vi "HFRR ADV v09.vi"() -> ()   [LabVIEW 2025] (continued)
                    n430 = local write "Main Dashboard Buttons"(T1."Home" ("Main Dashboard Buttons")) -> ()
                  }
                }
              }
              frame "Calibrate" {
              }
            }
          }
          frame #2 {
            n431 = Not(x=w709) -> (.not. x?=w708:bool)
            n432 = local write "Confirm Measrurement"(w708) -> ()
            n433 = local read "Calibration Tab"() -> (w707:enum32{"Measrument", "Calibrate"})
            n434 = case shown="\"Measrument\", Default" w707 {
              frame "Measrument", Default {
                n435 = local write "Main Tab"(T2."HOME" ("Main Tab")) -> ()
              }
              frame "Calibrate" {
              }
            }
          }
        }
      }
    }
    n436 = local read "Humidity"() -> (w462:bool)
    n437 = local read "Save Change"() -> (w467:bool)
    n438 = local read "Calibrate"() -> (w468:bool)
    n439 = local read "Auto Start Test"() -> (w463:bool)
    n440 = case shown="True" w468 {
      selector: w468 -> [_ w575]
      frame False {
      }
      frame True {
        n441 = Not(x=w575) -> (.not. x?=w574:bool)
        n442 = local write "Calibrate"(w574) -> ()
        n443 = local write "Calibration Tab"(enum32{"Measrument", "Calibrate"}."Calibrate" ("Calibration Tab")) -> ()
      }
    }
    n444 = case shown="True" w467 {
      selector: w467 -> [_ w519]
      frame False {
      }
      frame True {
        n445 = stacked-sequence {
          tunnel: w519 -> [_ _ _ _ w573]
          frame #0 {
            n446 = call "IMAGE ANALYSIS.vi"("Enum"=POST_ANALYSIS_ENUM."HIDE UI") -> ()  [unwired: 9 in, 2 out]
          }
          frame #1 {
            n447 = local read "100x gain"() -> (w521:dbl)
            n448 = local read "10x Gain"() -> (w522:dbl)
            n449 = local read "5x Gain"() -> (w523:dbl)
            n450 = Number To Fractional String(number=w522, width (-)=i16 4, precision (6)=i16 7) -> (F-format string=w544:string)  [unwired: 1 in]
            n451 = Number To Fractional String(number=0.0, width (-)=i16 4, precision (6)=i16 7) -> (F-format string=w539:string)  [unwired: 1 in]
            n452 = Number To Fractional String(number=w521, width (-)=i16 4, precision (6)=i16 7) -> (F-format string=w527:string)  [unwired: 1 in]
            n453 = Number To Fractional String(number=w523, width (-)=i16 10 ("precision (6)"), precision (6)=i16 7) -> (F-format string=w553:string)  [unwired: 1 in]
            n454 = Concatenate Strings("[CH1]" ("string"), w553, " - 5x Gain" ("string"), "\r") -> (w543:string)
            n455 = Concatenate Strings("[CH2]" ("string"), w544, " - 10x Gain" ("string"), "\r") -> (w542:string)
            n456 = Concatenate Strings("[CH3]" ("string"), w539, " - 20x Gain" ("string"), "\r") -> (w533:string)
            n457 = Concatenate Strings("[CH4]" ("string"), w527, " - 100x Gain" ("string"), "\r") -> (w526:string)
            n458 = String To Path(string="C:\\LAB-IQ\\Image Calibrate v01.dcf") -> (path=w556:path)
            n459 = Concatenate Strings(w543, w542, w533, w526) -> (w541:string)
            n460 = call <vilib>:"Write Characters To File.vi"("append to file? (new file:F)"=FALSE, "character string"=w541, "file path (dialog if empty)"=w556) -> ()  [unwired: 2 in, 1 out]
          }
          frame #2 {
            n461 = String To Path(string="C:\\LAB-IQ\\Image Calibrate v01.dcf") -> (path=w559:path)
            n462 = Open/Create/Replace File ("Open File")(file path (use dialog)=w559) -> (refnum out=w560:refnum<file>)  [unwired: 5 in, 2 out]
            n463 = for {
              N: 4 -> [_]
              tunnel: w560 -> [w566]
              i -> [w562]
              n464 = Read from Text File ("Read File")(file (use dialog)=w566) -> (text=w567:string)  [unwired: 3 in, 3 out]
              n465 = String Subset(string=w567, offset (0)=6, length (rest)=10 ("length (rest)")) -> (substring=w563:string)
              n466 = Fract/Exp String To Number(string=w563) -> (number=w561:dbl)  [unwired: 3 in, 1 out]
              n467 = case shown="3" w562 {
                tunnel: w561 -> [w568 w569 _ w570 _]
                frame 0 {
                  n468 = local write "5x Gain"(w568) -> ()
                }
                frame 1 {
                  n469 = local write "10x Gain"(w569) -> ()
                }
                frame 2 {
                }
                frame 3 {
                  n470 = local write "100x gain"(w570) -> ()
                }
                frame 4, Default {
                }
              }
            }
          }
          frame #3 {
            n471 = call "IMAGE ANALYSIS.vi"("Enum"=POST_ANALYSIS_ENUM."SHOW UI") -> ()  [unwired: 9 in, 2 out]
          }
          frame #4 {
            n472 = Not(x=w573) -> (.not. x?=w572:bool)
            n473 = local write "Save Change"(w572) -> ()
          }
        }
      }
    }
    n474 = case shown="False" w463 {
      tunnel: w462 -> [w489 _]
      frame False {
        n475 = case shown="True" w489 {
          frame False {
          }
          frame True {
            n476 = local read "Set Humidity:"() -> (w493:dbl)
            n477 = local read "Set Humidity:"() -> (w496:dbl)
            n478 = local read "Humidity ( %RH )"() -> (w497:dbl)
            n479 = Subtract(x=w493, y=1.0) -> (x-y=w491:dbl)
            n480 = Add(x=w496, y=1.0) -> (x+y=w492:dbl)
            n481 = In Range and Coerce(upper limit=w492, x=w497, lower limit=w491) -> (In Range?=w490:bool)  [unwired: 1 out]
            n482 = case shown="True" w490 {
              frame False {
              }
              frame True {
                n483 = case shown="True" "Manual Humididty Reached" {
                  selector: "Manual Humididty Reached" -> [_ w500]
                  frame False {
                  }
                  frame True {
                    n484 = Not(x=w500) -> (.not. x?=w499:bool)
                    n485 = local write "Manual Humididty Reached"(w499) -> ()
                    n486 = local read "EVENT LOG"() -> (w502:string)
                    n487 = call "Event Log.vi"("Content"="Target Humidity reached", "EVENT LOG"=w502) -> ("EVENT LOG"=w501:string)  [unwired: 8 in, 1 out]
                    n488 = local write "EVENT LOG"(w501) -> ()
                  }
                }
              }
            }
          }
        }
      }
      frame True {
        n489 = local write "Manual Humididty Reached"(TRUE ("Manual Humididty Reached")) -> ()
      }
    }
    n490 = local read "Cap Live Image"() -> (w483:bool)
    n491 = local read "SCAR MEASURMENT"() -> (w486:enum32{"Auto Scar", "Manual Scar"})
    n492 = Wait (ms)(milliseconds to wait=u32 250) -> ()  [unwired: 1 out]
    n493 = Equal?(x=w486, y=enum32{"Auto Scar", "Manual Scar"}."Manual Scar" ("SCAR MEASURMENT")) -> (x = y?=w484:bool)
    n494 = And(x=w484, y=w483) -> (x .and. y?=w482:bool)
    n495 = case shown="True" w482 {
      selector: w482 -> [_ w788]
      frame False {
      }
      frame True {
        n496 = stacked-sequence {
          tunnel: [_ _ _ w803 _] -> _
          tunnel: w788 -> [_ _ _ _ w809]
          frame #0 {
            w789 = 0.0
            n497 = local write "Major Axis"(w789) -> ()
            n498 = local write "Minor Axis"(w789) -> ()
            n499 = local write "Average"(w789) -> ()
          }
          frame #1 {
            n500 = call "CAMERA LIVE FEED FGV.vi"("Enum - Menu"=CAMERA_LIVE_FEED_ENUM."CAMERA MINIMIZE") -> ()  [unwired: 9 in, 2 out]
          }
          frame #2 {
            n501 = local read "FILE 3"() -> (w797:string)
            n502 = call <vilib>:"Trim Whitespace.vi"("string"="C:\\LAB-IQ\\images\\") -> ("trimmed string"=w799:string)  [unwired: 1 in]
            n503 = String To Path(string=w799) -> (path=w798:path)
            n504 = Concatenate Strings(w797, ".png" ("string")) -> (w796:string)
            n505 = Build Path(base path=w798, name or relative path=w796) -> (appended path=w794:path)
            n506 = Path To String(path=w794) -> (string=w793:string)
            n507 = call "CAMERA LIVE FEED FGV.vi"("Enum - Menu"=CAMERA_LIVE_FEED_ENUM."CAMERA SAVE", "Image Path"=w793) -> ("error out"=w791:errorcluster)  [unwired: 8 in, 1 out]
            n508 = case shown="No Error" w791 {
              frame No Error {
                n509 = One Button Dialog(message="Image saved successfully") -> ()  [unwired: 1 in, 1 out]
              }
              frame Error {
              }
            }
          }
          frame #3 {
            n510 = call "LIST FILE NAMES.vi"() -> ("error out"=w805:errorcluster, "filenames"=w802:string[])  [unwired: 10 in]
            n511 = call "IMAGE ANALYSIS.vi"("Enum"=POST_ANALYSIS_ENUM."SHOW UI", "error in"=w805) -> ("error out"=w803:errorcluster)  [unwired: 8 in, 1 out]
            n512 = property on="Test File List :" class="CmbBox"("Strings[]"=w802) -> ()  [unwired: 2 in, 2 out]
          }
          frame #4 {
            (unwired) T21."Report" ("Main Dashboard Buttons")
            n513 = Not(x=w809) -> (.not. x?=w808:bool)
            n514 = local write "Zoom Factore"(0.0 ("Zoom Factore")) -> ()
            n515 = local write "Cap Live Image"(w808) -> ()
            n516 = local write "Main Tab"(T2."Adv Scar Report" ("Main Tab")) -> ()
            n517 = property on="Cap Live Image" class="Bool (strict)"("BoolText.Text"="Capture Image" ("Boolean Text.Text")) -> ()  [unwired: 2 in, 2 out]
            n518 = local write "Main Dashboard Buttons"(T1."Report" ("Main Dashboard Buttons")) -> ()
          }
        }
      }
    }
    n519 = local read "change Gain"() -> (w466:bool)
    n520 = local read "Back Square"() -> (w465:bool)
    n521 = case shown="True" w466 {
      selector: w466 -> [_ w510]
      frame False {
      }
      frame True {
        n522 = stacked-sequence {
          tunnel: w510 -> [_ w518]
          frame #0 {
            n523 = local read "Actual (µm)"() -> (w514:dbl)
            n524 = local read "Pixel Value"() -> (w513:dbl)
            n525 = local read "Magnification :"() -> (w512:string)
            n526 = Divide(x=w514, y=w513) -> (x/y=w511:dbl)
            n527 = case shown="\"10x\"" w512 {
              tunnel: w511 -> [w515 w516]
              frame "10x" {
                n528 = local write "10x Gain"(w515) -> ()
              }
              frame "5x", Default {
                n529 = local write "5x Gain"(w516) -> ()
              }
            }
          }
          frame #1 {
            n530 = Not(x=w518) -> (.not. x?=w517:bool)
            n531 = local write "change Gain"(w517) -> ()
          }
        }
      }
    }
    n532 = case shown="True" w465 {
      selector: w465 -> [_ w508]
      frame False {
      }
      frame True {
        n533 = Not(x=w508) -> (.not. x?=w507:bool)
        n534 = local write "Back Square"(w507) -> ()
        n535 = local write "Calibration Tab"(enum32{"Measrument", "Calibrate"}."Measrument" ("Calibration Tab")) -> ()
      }
    }
    n536 = local read "Rectangle Tool"() -> (w477:bool)
    n537 = local read "Clear ROI Tool"() -> (w476:bool)
    n538 = local read "Open Image"() -> (w481:bool)
    n539 = local read "line tool"() -> (w478:bool)
    n540 = local read "OUT"() -> (w479:bool)
    n541 = local read "In"() -> (w480:bool)
    n542 = case shown="True" w481 {
      selector: w481 -> [_ w776]
      tunnel: [w772 w778] -> _
      tunnel: w471 -> [w772 w777]
      frame False {
      }
      frame True {
        n543 = Not(x=w776) -> (.not. x?=w775:bool)
        n544 = local write "Open Image"(w775) -> ()
        n545 = call "IMAGE ANALYSIS.vi"("Enum"=POST_ANALYSIS_ENUM."HIDE UI", "error in"=w777) -> ("error out"=w785:errorcluster)  [unwired: 8 in, 1 out]
        n546 = call "File Dialog"("start path"=path "C:/LAB-IQ/images", "error in"=w785) -> ("selected path"=w774:path, "error out"=w783:errorcluster)  [unwired: 10 in, 2 out]
        "Image path  2" <- w774
        n547 = call <vilib>:"Clear Errors.vi"("error in (no error)"=w783) -> ("error out"=w782:errorcluster)  [unwired: 5 in, 1 out]
        n548 = call "IMAGE ANALYSIS.vi"("Enum"=POST_ANALYSIS_ENUM."OPEN FILE", "error in"=w782, "File Path"=w774) -> ("error out"=w781:errorcluster)  [unwired: 7 in, 1 out]
        n549 = call <vilib>:"Clear Errors.vi"("error in (no error)"=w781) -> ("error out"=w780:errorcluster)  [unwired: 5 in, 1 out]
        n550 = call "IMAGE ANALYSIS.vi"("Enum"=POST_ANALYSIS_ENUM."SHOW UI", "error in"=w780) -> ("error out"=w778:errorcluster)  [unwired: 8 in, 1 out]
        n551 = local write "Zoom Factore"(100.0 ("Zoom Factore")) -> ()
      }
    }
    n552 = case shown="True" w479 {
      selector: w479 -> [_ w757]
      tunnel: w471 -> [w754 w762]
      tunnel: [w754 w756] -> _
      frame False {
      }
      frame True {
        n553 = Not(x=w757) -> (.not. x?=w755:bool)
        n554 = local read "Zoom Factore"() -> (w760:dbl)
        n555 = local write "OUT"(w755) -> ()
        n556 = call "IMAGE ANALYSIS.vi"("Enum"=POST_ANALYSIS_ENUM."ZOOM OUT", "error in"=w762) -> ("error out"=w756:errorcluster)  [unwired: 8 in, 1 out]
        n557 = Divide(x=w760, y=1.2) -> (x/y=w758:dbl)
        n558 = local write "Zoom Factore"(w758) -> ()
      }
    }
    n559 = case shown="True" w480 {
      selector: w480 -> [_ w766]
      tunnel: w471 -> [w763 w771]
      tunnel: [w763 w764] -> _
      frame False {
      }
      frame True {
        n560 = Not(x=w766) -> (.not. x?=w765:bool)
        n561 = local read "Zoom Factore"() -> (w769:dbl)
        n562 = local write "In"(w765) -> ()
        n563 = call "IMAGE ANALYSIS.vi"("Enum"=POST_ANALYSIS_ENUM."ZOOM IN", "error in"=w771) -> ("error out"=w764:errorcluster)  [unwired: 8 in, 1 out]
        n564 = Multiply(x=w769, y=1.2) -> (x*y=w767:dbl)
        n565 = local write "Zoom Factore"(w767) -> ()
      }
    }
    n566 = case shown="True" w476 {
      selector: w476 -> [_ w738]
      tunnel: w471 -> [w736 w740]
      tunnel: [w736 w739] -> _
      frame False {
      }
      frame True {
        n567 = Not(x=w738) -> (.not. x?=w737:bool)
        n568 = local write "Clear ROI Tool"(w737) -> ()
        n569 = call "IMAGE ANALYSIS.vi"("Enum"=POST_ANALYSIS_ENUM."CLEAR ROI", "error in"=w740) -> ("error out"=w739:errorcluster)  [unwired: 8 in, 1 out]
      }
    }
    n570 = case shown="True" w478 {
      selector: w478 -> [_ w750]
      tunnel: w471 -> [w748 w753]
      tunnel: [w748 w751] -> _
      frame False {
      }
      frame True {
        n571 = Not(x=w750) -> (.not. x?=w749:bool)
        n572 = local write "line tool"(w749) -> ()
        n573 = call "IMAGE ANALYSIS.vi"("Enum"=POST_ANALYSIS_ENUM."DRAW LINE", "error in"=w753) -> ("error out"=w751:errorcluster)  [unwired: 8 in, 1 out]
      }
    }
    n574 = case shown="True" w477 {
      selector: w477 -> [_ w744]
      tunnel: w471 -> [w742 w746]
      tunnel: [w742 w745] -> _
      frame False {
      }
      frame True {
        n575 = Not(x=w744) -> (.not. x?=w743:bool)
        n576 = local write "Rectangle Tool"(w743) -> ()
        n577 = call "IMAGE ANALYSIS.vi"("Enum"=POST_ANALYSIS_ENUM."DRAW REC", "error in"=w746) -> ("error out"=w745:errorcluster)  [unwired: 8 in, 1 out]
      }
    }
    n578 = local read "SCAR MEASURMENT"() -> (w464:enum32{"Auto Scar", "Manual Scar"})
    n579 = local read "Fit to Screen Tool"() -> (w473:bool)
    n580 = local read "Resize Tool"() -> (w472:bool)
    n581 = case shown="\"Manual Scar\"" w464 {
      frame "Auto Scar", Default {
        n582 = property on="Cap Live Image" class="Bool (strict)"("BoolText.Text"="Report" ("Boolean Text.Text")) -> ()  [unwired: 2 in, 2 out]
      }
      frame "Manual Scar" {
        n583 = property on="Cap Live Image" class="Bool (strict)"("BoolText.Text"="Save Image" ("Boolean Text.Text")) -> ()  [unwired: 2 in, 2 out]
      }
    }
    n584 = local read "ROI Color Tool"() -> (w474:bool)
    n585 = local read "Pan Tool"() -> (w475:bool)
    n586 = case shown="True" w475 {
      selector: w475 -> [_ w732]
      tunnel: w471 -> [w730 w734]
      tunnel: [w730 w733] -> _
      frame False {
      }
      frame True {
        n587 = Not(x=w732) -> (.not. x?=w731:bool)
        n588 = call "IMAGE ANALYSIS.vi"("Enum"=POST_ANALYSIS_ENUM."PAN", "error in"=w734) -> ("error out"=w733:errorcluster)  [unwired: 8 in, 1 out]
        n589 = local write "Pan Tool"(w731) -> ()
      }
    }
    n590 = case shown="True" w472 {
      selector: w472 -> [_ w716]
      tunnel: w471 -> [w711 w713]
      tunnel: [w711 w712] -> _
      frame False {
      }
      frame True {
        n591 = Not(x=w716) -> (.not. x?=w715:bool)
        n592 = local write "Resize Tool"(w715) -> ()
        n593 = call "IMAGE ANALYSIS.vi"("Enum"=POST_ANALYSIS_ENUM."RESIZE MODE", "error in"=w713) -> ("error out"=w712:errorcluster)  [unwired: 8 in, 1 out]
      }
    }
    n594 = case shown="True" w473 {
      selector: w473 -> [_ w721]
      tunnel: [w717 w722] -> _
      tunnel: w471 -> [w717 w720]
      frame False {
      }
      frame True {
        n595 = Not(x=w721) -> (.not. x?=w719:bool)
        n596 = local write "Zoom Factore"(100.0 ("Zoom Factore")) -> ()
        n597 = local write "Fit to Screen Tool"(w719) -> ()
        n598 = call "IMAGE ANALYSIS.vi"("Enum"=POST_ANALYSIS_ENUM."FIT", "error in"=w720) -> ("error out"=w722:errorcluster)  [unwired: 8 in, 1 out]
      }
    }
    n599 = case shown="True" w474 {
      selector: w474 -> [_ w727]
      tunnel: [w724 w728] -> _
      tunnel: w471 -> [w724 w725]
      frame False {
      }
      frame True {
        n600 = Not(x=w727) -> (.not. x?=w726:bool)
        n601 = local write "ROI Color Tool"(w726) -> ()
        n602 = call "IMAGE ANALYSIS.vi"("Enum"=POST_ANALYSIS_ENUM."SET ROI COLOR", "error in"=w725) -> ("error out"=w728:errorcluster)  [unwired: 8 in, 1 out]
      }
    }
    n603 = local read "Quit"() -> (w488:bool)
  }
  n604 = local write "USERNAME"(w23) -> ()
  n605 = local write "Main Tab"(T2."HOME" ("Main Tab")) -> ()
  n606 = local write "USER ID"(w23) -> ()
  n607 = property on="Auto Scar Check  2" class="Clust (strict)"("Visible"=w4) -> (error out=w8:errorcluster)  [unwired: 2 in, 1 out]
  n608 = property on="Quit" class="Bool (strict)"("Value"=FALSE ("Quit")) -> (error out=w25:errorcluster)  [unwired: 2 in, 1 out]
  n609 = while {
    stop <- w812 stop-if-true
    n610 = local read "Image Path"() -> (w815:path)
    n611 = local read "Print 3"() -> (w818:bool)
    n612 = Equal?(x=w815, y=path "") -> (x = y?=w814:bool)
    n613 = Not(x=w814) -> (.not. x?=w813:bool)
    n614 = property on="Print 3" class="Bool (strict)"("Visible"=w813) -> ()  [unwired: 2 in, 2 out]
    n615 = case shown="True" w818 {
      frame False {
        n616 = local write "Rd"(TRUE ("Boolean 7")) -> ()
      }
      frame True {
        n617 = flat-sequence {
          tunnel: [w858] -> w826
          tunnel: [w845] -> w824
          tunnel: [w855] -> w820
          tunnel: w826 -> [w867]
          tunnel: [w867] -> w825
          tunnel: w824 -> [w866]
          tunnel: [w866] -> w823
          tunnel: [w864] -> w822
          tunnel: [w863] -> w821
          tunnel: w820 -> [w863]
          tunnel: w825 -> [w869]
          tunnel: w823 -> [w870]
          tunnel: w822 -> [_]
          tunnel: w821 -> [w868]
          frame #0 {
            n618 = case shown="True" "Rd" {
              frame False {
              }
              frame True {
                n619 = while {
                  tunnel: "abcdefABCDEF" ("string 2") -> [w837]
                  shift-right: [w835] -> w829
                  shift-left: "" -> [w834]
                  i -> [w844]
                  stop <- w843 stop-if-true
                  n620 = Random Number (0-1)() -> (number: 0 to 1=w838:dbl)
                  n621 = Multiply(x=w838, y=62.0) -> (x*y=w840:dbl)
                  n622 = Decrement(x="Length 2") -> (x-1=w833:i16)
                  n623 = To Word Integer(number=w840) -> (16bit integer=w841:i16)
                  n624 = String Subset(string=w837, offset (0)=w841, length (rest)=1 ("length (rest)")) -> (substring=w836:string)
                  n625 = Greater Or Equal?(x=w844, y=w833) -> (x >= y?=w843:bool)
                  n626 = Concatenate Strings(w836, w834) -> (w835:string)
                }
                "String 10" <- w829
                n627 = local write "Rd"(FALSE ("Boolean 7")) -> ()
              }
            }
          }
          frame #1 {
            w856 = "_resized.jpg" ("command line")
            (unwired) ".jpg -resize 320x240 " ("string")
            (unwired) "Choose an Image File" ("prompt")
            # "-resize 1798x425"
            n628 = local read "Image Path"() -> (w850:path)
            n629 = Strip Path(path=w850) -> (stripped path=w845:path, name=w846:string)
            n630 = Match Pattern(string=w846, regular expression=".jpg") -> (before substring=→"before substring 2":string, after substring=→"after substring":string)  [unwired: 1 in, 2 out]
            n631 = Match Pattern(string=w846, regular expression="\\") -> (before substring=w852:string)  [unwired: 1 in, 3 out]
            n632 = Match Pattern(string=w852, regular expression=".jpg") -> (before substring=w851:string)  [unwired: 1 in, 3 out]
            n633 = Concatenate Strings("cmd /c convert " ("string"), w851, ".jpg -resize 320x240  " ("command line"), w851, w856) -> (w859:string)
            n634 = call <vilib>:"System Exec.vi"("run minimized? (F)"=TRUE, "wait until completion? (T)"=TRUE, "working directory"=w845, "command line"=w859) -> ("error out"=w858:errorcluster)  [unwired: 4 in, 3 out]
            "error out 2" <- w858
            n635 = Concatenate Strings(w851, w856) -> (w855:string)
          }
          frame #2 {
            n636 = Wait (ms)(milliseconds to wait=u32 2000 ("millisecond timer value")) -> (millisecond timer value=w864:u32)
          }
          frame #3 {
            n637 = case shown="No Error" w869 {
              tunnel: w870 -> [w873 _]
              tunnel: w868 -> [w871 _]
              frame No Error {
                (unwired) ".jpg" ("string")
                n638 = Path To String(path=w873) -> (string=w877:string)
                n639 = Concatenate Strings(w877, "\\" ("string"), w871) -> (w876:string)
                n640 = String To Path(string=w876) -> (path=w875:path)
                n641 = call <vilib>:"Read JPEG File.vi"("path to JPEG file"=w875) -> ("image data"=w879:T13)  [unwired: 8 in, 2 out]
                "image data" <- w879
                n642 = local write "Print 3"(FALSE ("Print 2")) -> ()
                n643 = call <vilib>:"Draw Flattened Pixmap.vi"("image data"=w879) -> ("new picture"=→"new picture":picture)  [unwired: 8 in]
              }
              frame Error {
              }
            }
          }
        }
      }
    }
    n644 = Wait (ms)(milliseconds to wait=u32 20 ("millisecond timer value")) -> ()  [unwired: 1 out]
    n645 = local read "Quit"() -> (w812:bool)
  }
  n646 = property on="Service Password Log" class="Str"("Visible"=w4) -> ()  [unwired: 2 in, 2 out]
  n647 = property on="Password 3" class="Clust (strict)"("Visible"=w4) -> ()  [unwired: 2 in, 2 out]
  n648 = while {
    tunnel: w25 -> [_]
    tunnel: w8 -> [_]
    stop <- w910 stop-if-true
    # "New Adv Logics"
    n649 = local read "Main Tab"() -> (w908:T2)
    n650 = local read "Sign In"() -> (w907:bool)
    n651 = local read "Main Tab"() -> (w889:T2)
    n652 = case shown="\"About\"" w889 {
      frame "HOME", Default {
        n653 = local read "LIVE FEED MIN TEMP"() -> (w1032:bool)
        n654 = local write "LIVE FEED MAX TEMP"(TRUE ("LIVE FEED MAX TEMP")) -> ()
        n655 = local read "CAMERA ROI MIN TEMP"() -> (w1030:bool)
        n656 = case shown="True" w1032 {
          selector: w1032 -> [_ w1039]
          frame False {
          }
          frame True {
            n657 = Not(x=w1039) -> (.not. x?=w1038:bool)
            n658 = local write "LIVE FEED MIN TEMP"(w1038) -> ()
            n659 = call "CAMERA LIVE FEED FGV.vi"("Enum - Menu"=CAMERA_LIVE_FEED_ENUM."CAMERA MINIMIZE") -> ()  [unwired: 9 in, 2 out]
          }
        }
        n660 = case shown="True" w1030 {
          selector: w1030 -> [_ w1036]
          frame False {
          }
          frame True {
            n661 = Not(x=w1036) -> (.not. x?=w1035:bool)
            n662 = local write "CAMERA ROI MIN TEMP"(w1035) -> ()
            n663 = call "IMAGE ANALYSIS.vi"("Enum"=POST_ANALYSIS_ENUM."MINIMIZE UI") -> ()  [unwired: 9 in, 2 out]
          }
        }
        n664 = local write "CAMERA ROI MAX TEMP"(TRUE ("CAMERA ROI MAX TEMP")) -> ()
      }
      frame "Test Setup" {
        n665 = local read "LIVE FEED MIN TEMP"() -> (w1042:bool)
        n666 = local read "CAMERA ROI MIN TEMP"() -> (w1040:bool)
        n667 = local write "LIVE FEED MAX TEMP"(TRUE ("LIVE FEED MAX TEMP")) -> ()
        n668 = case shown="True" w1042 {
          selector: w1042 -> [_ w1049]
          frame False {
          }
          frame True {
            n669 = Not(x=w1049) -> (.not. x?=w1048:bool)
            n670 = local write "LIVE FEED MIN TEMP"(w1048) -> ()
            n671 = call "CAMERA LIVE FEED FGV.vi"("Enum - Menu"=CAMERA_LIVE_FEED_ENUM."CAMERA MINIMIZE") -> ()  [unwired: 9 in, 2 out]
          }
        }
        n672 = case shown="True" w1040 {
          selector: w1040 -> [_ w1046]
          frame False {
          }
          frame True {
            n673 = Not(x=w1046) -> (.not. x?=w1045:bool)
            n674 = local write "CAMERA ROI MIN TEMP"(w1045) -> ()
            n675 = call "IMAGE ANALYSIS.vi"("Enum"=POST_ANALYSIS_ENUM."MINIMIZE UI") -> ()  [unwired: 9 in, 2 out]
          }
        }
        n676 = local write "CAMERA ROI MAX TEMP"(TRUE ("CAMERA ROI MAX TEMP")) -> ()
      }
      frame "Acquire" {
        n677 = local read "LIVE FEED MIN TEMP"() -> (w1052:bool)
        n678 = local write "LIVE FEED MAX TEMP"(TRUE ("LIVE FEED MAX TEMP")) -> ()
        n679 = local read "CAMERA ROI MIN TEMP"() -> (w1050:bool)
        n680 = case shown="True" w1052 {
          selector: w1052 -> [_ w1059]
          frame False {
          }
          frame True {
            n681 = Not(x=w1059) -> (.not. x?=w1058:bool)
            n682 = local write "LIVE FEED MIN TEMP"(w1058) -> ()
            n683 = call "CAMERA LIVE FEED FGV.vi"("Enum - Menu"=CAMERA_LIVE_FEED_ENUM."CAMERA MINIMIZE") -> ()  [unwired: 9 in, 2 out]
          }
        }
        n684 = case shown="True" w1050 {
          selector: w1050 -> [_ w1056]
          frame False {
          }
          frame True {
            n685 = Not(x=w1056) -> (.not. x?=w1055:bool)
            n686 = local write "CAMERA ROI MIN TEMP"(w1055) -> ()
            n687 = call "IMAGE ANALYSIS.vi"("Enum"=POST_ANALYSIS_ENUM."MINIMIZE UI") -> ()  [unwired: 9 in, 2 out]
          }
        }
        n688 = local write "CAMERA ROI MAX TEMP"(TRUE ("CAMERA ROI MAX TEMP")) -> ()
      }
      frame "Adv Scar" {
        n689 = local read "CAMERA ROI MIN TEMP"() -> (w1060:bool)
        n690 = case shown="True" "LIVE FEED MAX TEMP" {
          selector: "LIVE FEED MAX TEMP" -> [_ w1072]
          frame False {
          }
          frame True {
            n691 = Not(x=w1072) -> (.not. x?=w1071:bool)
            n692 = local write "LIVE FEED MAX TEMP"(w1071) -> ()
            n693 = call "CAMERA LIVE FEED FGV.vi"("Enum - Menu"=CAMERA_LIVE_FEED_ENUM."CAMERA RESTORE") -> ("error out"=w1067:errorcluster)  [unwired: 9 in, 1 out]
            n694 = call "LIST FILE NAMES.vi"("error in (no error)"=w1067) -> ("error out"=w1068:errorcluster, "filenames"=w1069:string[])  [unwired: 9 in]
            n695 = property on="FILE 3" class="CmbBox"(error in=w1068, "Strings[]"=w1069) -> ()  [unwired: 1 in, 2 out]
          }
        }
        n696 = case shown="True" w1060 {
          selector: w1060 -> [_ w1066]
          frame False {
          }
          frame True {
            n697 = Not(x=w1066) -> (.not. x?=w1065:bool)
            n698 = local write "CAMERA ROI MIN TEMP"(w1065) -> ()
            n699 = call "IMAGE ANALYSIS.vi"("Enum"=POST_ANALYSIS_ENUM."MINIMIZE UI") -> ()  [unwired: 9 in, 2 out]
          }
        }
        n700 = local write "CAMERA ROI MAX TEMP"(TRUE ("CAMERA ROI MAX TEMP")) -> ()
        "LIVE FEED MIN TEMP" <- TRUE ("LIVE FEED MIN TEMP")
      }
      frame "Adv Scar Report" {
        n701 = local read "CAMERA ROI MAX TEMP"() -> (w1073:bool)
        n702 = local read "LIVE FEED MIN TEMP"() -> (w1075:bool)
        n703 = local write "LIVE FEED MAX TEMP"(TRUE ("LIVE FEED MAX TEMP")) -> ()
        n704 = case shown="True" w1075 {
          selector: w1075 -> [_ w1084]
          frame False {
          }
          frame True {
            n705 = Not(x=w1084) -> (.not. x?=w1083:bool)
            n706 = local write "LIVE FEED MIN TEMP"(w1083) -> ()
            n707 = call "CAMERA LIVE FEED FGV.vi"("Enum - Menu"=CAMERA_LIVE_FEED_ENUM."CAMERA MINIMIZE") -> ()  [unwired: 9 in, 2 out]
          }
        }
        n708 = case shown="True" w1073 {
          selector: w1073 -> [_ w1081]
          frame False {
          }
          frame True {
            n709 = Not(x=w1081) -> (.not. x?=w1079:bool)
            n710 = local write "CAMERA ROI MAX TEMP"(w1079) -> ()
            n711 = call "IMAGE ANALYSIS.vi"("Enum"=POST_ANALYSIS_ENUM."SHOW UI") -> ("error out"=w1078:errorcluster)  [unwired: 9 in, 1 out]
            n712 = call "LIST FILE NAMES.vi"("error in (no error)"=w1078) -> ("filenames"=w1077:string[])  [unwired: 9 in, 1 out]
            n713 = property on="Test File List :" class="CmbBox"("Strings[]"=w1077) -> ()  [unwired: 2 in, 2 out]
          }
        }
        n714 = local write "CAMERA ROI MIN TEMP"(TRUE ("CAMERA ROI MIN TEMP")) -> ()
      }
      frame "Compare Files" {
        n715 = local read "LIVE FEED MIN TEMP"() -> (w1087:bool)
        n716 = local write "LIVE FEED MAX TEMP"(TRUE ("LIVE FEED MAX TEMP")) -> ()
        n717 = local read "CAMERA ROI MIN TEMP"() -> (w1085:bool)
        n718 = case shown="True" w1087 {
          selector: w1087 -> [_ w1094]
          frame False {
          }
          frame True {
            n719 = Not(x=w1094) -> (.not. x?=w1093:bool)
            n720 = local write "LIVE FEED MIN TEMP"(w1093) -> ()
            n721 = call "CAMERA LIVE FEED FGV.vi"("Enum - Menu"=CAMERA_LIVE_FEED_ENUM."CAMERA MINIMIZE") -> ()  [unwired: 9 in, 2 out]
          }
        }
        n722 = case shown="True" w1085 {
          selector: w1085 -> [_ w1091]
          frame False {
          }
          frame True {
            n723 = Not(x=w1091) -> (.not. x?=w1090:bool)
            n724 = local write "CAMERA ROI MIN TEMP"(w1090) -> ()
            n725 = call "IMAGE ANALYSIS.vi"("Enum"=POST_ANALYSIS_ENUM."MINIMIZE UI") -> ()  [unwired: 9 in, 2 out]
          }
        }
        n726 = local write "CAMERA ROI MAX TEMP"(TRUE ("CAMERA ROI MAX TEMP")) -> ()
      }
      frame "About" {
        n727 = local read "LIVE FEED MIN TEMP"() -> (w1097:bool)
        n728 = local write "LIVE FEED MAX TEMP"(TRUE ("LIVE FEED MAX TEMP")) -> ()
        n729 = local read "CAMERA ROI MIN TEMP"() -> (w1096:bool)
        n730 = case shown="True" w1097 {
          selector: w1097 -> [_ w1104]
          frame False {
          }
          frame True {
            n731 = Not(x=w1104) -> (.not. x?=w1103:bool)
            n732 = local write "LIVE FEED MIN TEMP"(w1103) -> ()
            n733 = call "CAMERA LIVE FEED FGV.vi"("Enum - Menu"=CAMERA_LIVE_FEED_ENUM."CAMERA MINIMIZE") -> ()  [unwired: 9 in, 2 out]
          }
        }
        n734 = case shown="True" w1096 {
          selector: w1096 -> [_ w1101]
          frame False {
          }
          frame True {
            n735 = Not(x=w1101) -> (.not. x?=w1100:bool)
            n736 = local write "CAMERA ROI MIN TEMP"(w1100) -> ()
            n737 = call "IMAGE ANALYSIS.vi"("Enum"=POST_ANALYSIS_ENUM."MINIMIZE UI") -> ()  [unwired: 9 in, 2 out]
          }
        }
        n738 = local write "CAMERA ROI MAX TEMP"(TRUE ("CAMERA ROI MIN TEMP")) -> ()
      }
      frame "Advance" {
        n739 = local read "LIVE FEED MIN TEMP"() -> (w1107:bool)
        n740 = local write "LIVE FEED MAX TEMP"(TRUE ("LIVE FEED MAX TEMP")) -> ()
        n741 = local read "CAMERA ROI MIN TEMP"() -> (w1105:bool)
        n742 = case shown="True" w1107 {
          selector: w1107 -> [_ w1114]
          frame False {
          }
          frame True {
            n743 = Not(x=w1114) -> (.not. x?=w1113:bool)
            n744 = local write "LIVE FEED MIN TEMP"(w1113) -> ()
            n745 = call "CAMERA LIVE FEED FGV.vi"("Enum - Menu"=CAMERA_LIVE_FEED_ENUM."CAMERA MINIMIZE") -> ()  [unwired: 9 in, 2 out]
          }
        }
        n746 = local write "CAMERA ROI MAX TEMP"(TRUE ("CAMERA ROI MAX TEMP")) -> ()
        n747 = case shown="True" w1105 {
          selector: w1105 -> [_ w1111]
          frame False {
          }
          frame True {
            n748 = Not(x=w1111) -> (.not. x?=w1110:bool)
            n749 = local write "CAMERA ROI MIN TEMP"(w1110) -> ()
            n750 = call "IMAGE ANALYSIS.vi"("Enum"=POST_ANALYSIS_ENUM."MINIMIZE UI") -> ()  [unwired: 9 in, 2 out]
          }
        }
      }
      frame "Mooha" {
        n751 = local read "LIVE FEED MIN TEMP"() -> (w1117:bool)
        n752 = local write "LIVE FEED MAX TEMP"(TRUE ("LIVE FEED MAX TEMP")) -> ()
        n753 = local read "CAMERA ROI MIN TEMP"() -> (w1115:bool)
        n754 = case shown="True" w1117 {
          selector: w1117 -> [_ w1124]
          frame False {
          }
          frame True {
            n755 = Not(x=w1124) -> (.not. x?=w1123:bool)
            n756 = local write "LIVE FEED MIN TEMP"(w1123) -> ()
            n757 = call "CAMERA LIVE FEED FGV.vi"("Enum - Menu"=CAMERA_LIVE_FEED_ENUM."CAMERA MINIMIZE") -> ()  [unwired: 9 in, 2 out]
          }
        }
        n758 = local write "CAMERA ROI MAX TEMP"(TRUE ("CAMERA ROI MAX TEMP")) -> ()
        n759 = case shown="True" w1115 {
          selector: w1115 -> [_ w1121]
          frame False {
          }
          frame True {
            n760 = Not(x=w1121) -> (.not. x?=w1120:bool)
            n761 = local write "CAMERA ROI MIN TEMP"(w1120) -> ()
            n762 = call "IMAGE ANALYSIS.vi"("Enum"=POST_ANALYSIS_ENUM."MINIMIZE UI") -> ()  [unwired: 9 in, 2 out]
          }
        }
      }
    }
    n763 = local read "Auto Start Test"() -> (w880:bool)
    n764 = case shown="True" "sign in temp" {
      frame False {
      }
      frame True {
        w917 = 1 ("y")
        n765 = local read "USERNAME"() -> (w923:string)
        n766 = local read "USER ID"() -> (w920:string)
        n767 = call <vilib>:"Trim Whitespace.vi"("string"=w923) -> ("trimmed string"=w922:string)  [unwired: 1 in]
        n768 = call <vilib>:"Trim Whitespace.vi"("string"=w920) -> ("trimmed string"=w921:string)  [unwired: 1 in]
        n769 = String Length(string=w922) -> (length=w919:i32)
        n770 = String Length(string=w921) -> (length=w918:i32)
        n771 = Greater?(x=w919, y=w917) -> (0:w916:bool)
        n772 = Greater?(x=w918, y=w917) -> (0:w915:bool)
        n773 = And(x=w916, y=w915) -> (x .and. y?=w914:bool)
        n774 = case shown="True" w914 {
          frame False {
            n775 = property on="Sign In" class="Bool (strict)"("DisabledEnum"=T15."Disabled" ("Disabled")) -> ()  [unwired: 2 in, 2 out]
          }
          frame True {
            n776 = property on="Sign In" class="Bool (strict)"("DisabledEnum"=T15."Enabled" ("Disabled")) -> ()  [unwired: 2 in, 2 out]
          }
        }
      }
    }
    n777 = local read "Air Temperature"() -> (w897:bool)
    n778 = local read "Coefficient Of Friction"() -> (w898:bool)
    n779 = case shown="False" w880 {
      frame False {
        n780 = local read "Auto stop temp"() -> (w911:bool)
        n781 = case shown="True" w911 {
          frame False {
          }
          frame True {
            n782 = local write "Auto Start Temp"(FALSE ("Auto Start Temp")) -> ()
          }
        }
      }
      frame True {
        "Auto stop temp" <- TRUE ("Auto stop temp")
      }
    }
    n783 = local read "Humidity"() -> (w896:bool)
    n784 = case shown="\"HOME\"" w908 {
      frame "HOME" {
        n785 = local write "main tab sub"(enum32{"Page 1", "Page 2"}."Page 1" ("main tab sub")) -> ()
      }
      frame Default {
        n786 = local write "main tab sub"(enum32{"Page 1", "Page 2"}."Page 2" ("main tab sub")) -> ()
      }
    }
    n787 = case shown="True" w907 {
      selector: w907 -> [_ w1214]
      frame False {
      }
      frame True {
        n788 = Not(x=w1214) -> (.not. x?=w1213:bool)
        n789 = local write "Sign In"(w1213) -> ()
        n790 = local write "Main Dashboard Buttons"(T1."Test Setup" ("Main Dashboard Buttons")) -> ()
      }
    }
    n791 = case shown="\"Numeric Display\", Default" "Num/Graph" {
      frame "Numeric Display", Default {
        n792 = property on="Single/Multiple" class="RadioBtnsControl (strict)"("Visible"=FALSE) -> ()  [unwired: 2 in, 2 out]
        n793 = property on="Single - Graph" class="Ring (strict)"("Visible"=FALSE) -> ()  [unwired: 2 in, 2 out]
        n794 = local write "Main Tab Display"(T4."Dashboard 1" ("Main Tab Display")) -> ()
      }
      frame "Graph Display" {
        n795 = property on="Single/Multiple" class="RadioBtnsControl (strict)"("Visible"=TRUE) -> ()  [unwired: 2 in, 2 out]
        n796 = case shown="\"Multiple\"" "Single/Multiple" {
          frame "Single ", Default {
            n797 = property on="Single - Graph" class="Ring (strict)"("Visible"=TRUE) -> ()  [unwired: 2 in, 2 out]
            n798 = local write "Main Tab Display"(T4."Dashboard 3" ("Main Tab Display")) -> ()
          }
          frame "Multiple" {
            n799 = property on="Single - Graph" class="Ring (strict)"("Visible"=FALSE) -> ()  [unwired: 2 in, 2 out]
            n800 = local write "Main Tab Display"(T4."Dashboard 2" ("Main Tab Display")) -> ()
          }
        }
      }
    }
    n801 = local read "Stroke"() -> (w895:bool)
    n802 = local read "USERNAME"() -> (w901:string)
    n803 = local read "USER ID"() -> (w900:string)
    n804 = case shown="True" w898 {
      selector: w898 -> [_ w1164]
      frame False {
      }
      frame True {
        n805 = Not(x=w1164) -> (.not. x?=w1163:bool)
        n806 = local write "Coefficient Of Friction"(w1163) -> ()
        n807 = local write "Tab Control 2"(T6."Coefficient Of Friction" ("Tab Control 2")) -> ()
      }
    }
    n808 = case shown="True" w897 {
      selector: w897 -> [_ w1161]
      frame False {
      }
      frame True {
        n809 = Not(x=w1161) -> (.not. x?=w1159:bool)
        n810 = local write "Air Temperature"(w1159) -> ()
        n811 = local write "Tab Control 2"(T6."Air Temperature" ("Tab Control 2")) -> ()
      }
    }
    n812 = local write "Operator ID"(w900) -> ()
    n813 = case shown="True" w895 {
      selector: w895 -> [_ w1155]
      frame False {
      }
      frame True {
        n814 = Not(x=w1155) -> (.not. x?=w1153:bool)
        n815 = local write "Stroke"(w1153) -> ()
        n816 = local write "Tab Control 2"(T6."Stroke" ("Tab Control 2")) -> ()
      }
    }
    n817 = local write "tested by"(w901) -> ()
    n818 = case shown="True" w896 {
      selector: w896 -> [_ w1158]
      frame False {
      }
      frame True {
        n819 = Not(x=w1158) -> (.not. x?=w1156:bool)
        n820 = local write "Humidity"(w1156) -> ()
        n821 = local write "Tab Control 2"(T6."Humidity" ("Tab Control 2")) -> ()
      }
    }
    n822 = case shown="\"Advance\"" "Main Dashboard Buttons" {
      tunnel: [T2."HOME" ("Main Tab") T2."Test Setup" ("Main Tab") T2."Acquire" ("Main Tab") T2."Adv Scar" ("Main Tab") T2."Adv Scar Report" ("Main Tab") T2."Compare Files" ("Main Tab") T2."About" ("Main Tab") T2."Advance" ("Main Tab")] -> w905
      frame "Home", Default {
      }
      frame "Test Setup" {
      }
      frame "Dashboard" {
      }
      frame "Imaging" {
      }
      frame "Report" {
      }
      frame "Analysis" {
      }
      frame "About" {
      }
      frame "Advance" {
      }
    }
    n823 = Wait (ms)(milliseconds to wait=u32 100) -> ()  [unwired: 1 out]
    n824 = local read "Main Tab Display"() -> (w899:T4)
    n825 = local write "Main Tab"(w905) -> ()
    n826 = case shown="\"Dashboard 3\"" w899 {
      frame "Dashboard 1", Default {
        n827 = property on="Reset Graph" class="Bool (strict)"("Visible"=FALSE) -> ()  [unwired: 2 in, 2 out]
      }
      frame "Dashboard 2" {
        n828 = property on="Reset Graph" class="Bool (strict)"("Visible"=TRUE) -> ()  [unwired: 2 in, 2 out]
      }
      frame "Dashboard 3" {
        n829 = property on="Reset Graph" class="Bool (strict)"("Visible"=TRUE) -> ()  [unwired: 2 in, 2 out]
      }
    }
    n830 = local read "SCAR MEASURMENT"() -> (w887:enum32{"Auto Scar", "Manual Scar"})
    n831 = local read "Humidity"() -> (w902:bool)
    n832 = local read "Cap Live Image"() -> (w884:bool)
    n833 = local read "Sample Temperature"() -> (w894:bool)
    n834 = local read "Air Temp vs Humidity"() -> (w892:bool)
    n835 = local read "Frequency"() -> (w893:bool)
    n836 = Equal?(x=w887, y=enum32{"Auto Scar", "Manual Scar"}."Auto Scar" ("SCAR MEASURMENT")) -> (x = y?=w883:bool)
    n837 = case shown="True" w902 {
      frame False {
        n838 = local write "Humidity On Command"(TRUE ("Humidity On Command")) -> ()
        n839 = case shown="True" "Humidity Off Command" {
          selector: "Humidity Off Command" -> [_ w1177]
          frame False {
          }
          frame True {
            n840 = Not(x=w1177) -> (.not. x?=w1176:bool)
            n841 = local write "Humidity Off Command"(w1176) -> ()
            n842 = local read "WriteHumidity"() -> (w1174:string[])
            n843 = local read "EVENT LOG"() -> (w1171:string)
            n844 = call "Event Log.vi"("Content"="Humidity Control Off" ("string"), "EVENT LOG"=w1171) -> ("EVENT LOG"=w1172:string)  [unwired: 8 in, 1 out]
            n845 = Insert Into Array(array=w1174, new element="R;1" ("new element/subarray")) -> (w1175:string[])  [unwired: 1 in]
            n846 = local write "EVENT LOG"(w1172) -> ()
            n847 = local write "WriteHumidity"(w1175) -> ()
          }
        }
      }
      frame True {
        n848 = case shown="True" "Humidity On Command" {
          selector: "Humidity On Command" -> [_ w1190]
          frame False {
          }
          frame True {
            n849 = local read "Set Rh"() -> (w1185:dbl)
            n850 = Not(x=w1190) -> (.not. x?=w1189:bool)
            n851 = local write "Humidity On Command"(w1189) -> ()
            n852 = Number To Fractional String(number=w1185, precision (6)=i16 2) -> (F-format string=w1182:string)  [unwired: 2 in]
            n853 = local read "WriteHumidity"() -> (w1187:string[])
            n854 = Concatenate Strings("M;" ("new element/subarray"), w1182) -> (w1186:string)
            n855 = Concatenate Strings("Humidity Set to : " ("string"), w1182, "% RH" ("string")) -> (w1180:string)
            n856 = Insert Into Array(array=w1187, new element=w1186) -> (w1188:string[])  [unwired: 1 in]
            n857 = disable-structure shown="Enabled" {
              disable-tunnel: w1180 -> [_ _]
              frame Enabled {
                n858 = local read "EVENT LOG"() -> (w1193:string)
                n859 = call "Event Log.vi"("Content"="Humidity Control On", "EVENT LOG"=w1193) -> ("EVENT LOG"=w1194:string)  [unwired: 8 in, 1 out]
                n860 = local write "EVENT LOG"(w1194) -> ()
              }
              frame Disabled {
              }
            }
            n861 = local write "WriteHumidity"(w1188) -> ()
          }
        }
        n862 = local write "Humidity Off Command"(TRUE ("Humidity Off Command")) -> ()
      }
    }
    n863 = local read "TEST STANDARD"() -> (w890:T3)
    n864 = And(x=w884, y=w883) -> (x .and. y?=w885:bool)
    n865 = case shown="True" w885 {
      selector: w885 -> [_ w983]
      tunnel: errorcluster {"status"=FALSE, "code"=0, "source"=""} ("error in (no error) 3") -> [_ w984]
      frame False {
      }
      frame True {
        n866 = stacked-sequence {
          tunnel: w984 -> [_ _ _ _ _ _ _ w1028]
          tunnel: w983 -> [_ _ _ _ _ w1011 _ _]
          frame #0 {
            n867 = call "CAMERA LIVE FEED FGV.vi"("Enum - Menu"=CAMERA_LIVE_FEED_ENUM."CAMERA MINIMIZE") -> ()  [unwired: 9 in, 2 out]
          }
          frame #1 {
            n868 = property on="Auto Scar Check  2" class="Clust (strict)"("Visible"=TRUE) -> ()  [unwired: 2 in, 2 out]
          }
          frame #2 {
            n869 = String To Path(string="C:\\LAB-IQ\\Image Calibrate v01.dcf") -> (path=w989:path)
            n870 = Open/Create/Replace File ("Open File")(file path (use dialog)=w989) -> (refnum out=w990:refnum<file>)  [unwired: 5 in, 2 out]
            n871 = for {
              N: 4 -> [_]
              tunnel: w990 -> [w996]
              i -> [w992]
              n872 = Read from Text File ("Read File")(file (use dialog)=w996) -> (text=w997:string)  [unwired: 3 in, 3 out]
              n873 = String Subset(string=w997, offset (0)=6, length (rest)=10 ("length (rest)")) -> (substring=w993:string)
              n874 = Fract/Exp String To Number(string=w993) -> (number=w991:dbl)  [unwired: 3 in, 1 out]
              n875 = case shown="0" w992 {
                tunnel: w991 -> [w998 w999 _ w1000 _]
                frame 0 {
                  "5x Gain" <- w998
                }
                frame 1 {
                  "10x Gain" <- w999
                }
                frame 2 {
                }
                frame 3 {
                  "100x gain" <- w1000
                }
                frame 4, Default {
                }
              }
            }
          }
          frame #3 {
            n876 = local read "FILE 3"() -> (w1006:string)
            n877 = call <vilib>:"Trim Whitespace.vi"("string"="C:\\LAB-IQ\\images\\") -> ("trimmed string"=w1008:string)  [unwired: 1 in]
            n878 = String To Path(string=w1008) -> (path=w1007:path)
            n879 = Concatenate Strings(w1006, ".png" ("string")) -> (w1005:string)
            n880 = Build Path(base path=w1007, name or relative path=w1005) -> (appended path=w1003:path)
            "Image path" <- w1003
            n881 = Path To String(path=w1003) -> (string=w1002:string)
            n882 = call "CAMERA LIVE FEED FGV.vi"("Enum - Menu"=CAMERA_LIVE_FEED_ENUM."CAMERA SAVE", "Image Path"=w1002) -> ()  [unwired: 8 in, 2 out]
          }
          frame #4 {
            n883 = One Button Dialog(message="Image saved successfully") -> ()  [unwired: 1 in, 1 out]
          }
          frame #5 {
            n884 = local read "Magnification len live scar"() -> (w1022:string)
            n885 = Not(x=w1011) -> (.not. x?=w1012:bool)
            n886 = local write "Cap Live Image"(w1012) -> ()
            n887 = case shown="\"5x\", Default" w1022 {
              tunnel: [w1023 w1024] -> w1021
              frame "5x", Default {
                n888 = local read "5x Gain"() -> (w1023:dbl)
              }
              frame "10x" {
                # "5x"
                n889 = local read "10x Gain"() -> (w1024:dbl)
              }
            }
            n890 = local read "Image path"() -> (w1020:path)
            n891 = local read "FILE 3"() -> (w1013:string)
            n892 = call "EDGE DETCTION.vi"("GAIN VALUE"=w1021, "Image Path"=w1020) -> ("error out"=w1019:errorcluster, "return value"=w1018:cluster{string, string, dbl, dbl, dbl})  [unwired: 8 in]
            n893 = Bundle By Name(cluster=T20 {"File Name"="", "Test Method"="", "Operator"="", "Fuel Description"="", "Date and time"=""} ("Main Ref"), "File Name"=w1013) -> (w1014:T20)
            n894 = call "duf file read.vi"("error in (no error)"=w1019, "Main Ref"=w1014) -> ("error out"=w1017:errorcluster, "Main Ref 2"=w1015:T20)  [unwired: 8 in]
            n895 = call "EDGE DETECTION REPORT.vi"("error in (no error)"=w1017, "return value 2"=w1018, "Main Ref"=w1015) -> ()  [unwired: 8 in, 1 out]
          }
          frame #6 {
            n896 = property on="Auto Scar Check  2" class="Clust (strict)"("Visible"=FALSE) -> ()  [unwired: 2 in, 2 out]
          }
          frame #7 {
            n897 = call "CAMERA LIVE FEED FGV.vi"("Enum - Menu"=CAMERA_LIVE_FEED_ENUM."CAMERA MINIMIZE", "error in (no error)"=w1028) -> ()  [unwired: 8 in, 2 out]
            n898 = local write "Main Dashboard Buttons"(T1."Home" ("Main Dashboard Buttons")) -> ()
            n899 = local write "Main Tab"(T2."HOME" ("Main Tab")) -> ()
          }
        }
      }
    }
    n900 = local read "Heater Button"() -> (w891:bool)
    n901 = case shown="True" w893 {
      selector: w893 -> [_ w1149]
      frame False {
      }
      frame True {
        n902 = Not(x=w1149) -> (.not. x?=w1147:bool)
        n903 = local write "Frequency"(w1147) -> ()
        n904 = local write "Tab Control 2"(T6."Frequency" ("Tab Control 2")) -> ()
      }
    }
    n905 = case shown="True" w892 {
      selector: w892 -> [_ w1146]
      frame False {
      }
      frame True {
        n906 = Not(x=w1146) -> (.not. x?=w1144:bool)
        n907 = local write "Air Temp vs Humidity"(w1144) -> ()
        n908 = local write "Tab Control 2"(T6."Air Temp vs Rh" ("Tab Control 2")) -> ()
      }
    }
    n909 = case shown="True" w894 {
      selector: w894 -> [_ w1152]
      frame False {
      }
      frame True {
        n910 = Not(x=w1152) -> (.not. x?=w1150:bool)
        n911 = local write "Sample Temperature"(w1150) -> ()
        n912 = local write "Tab Control 2"(T6."Sample Temperature" ("Tab Control 2")) -> ()
      }
    }
    n913 = case shown="\"Custom\"" w890 {
      frame "ASTM D6079", Default {
        w1125 = "ASTM D6079 TEST CONDITIONS" ("Standard 2")
        n914 = local write "Standard 2"(w1125) -> ()
        n915 = local write "Standard"(w1125) -> ()
      }
      frame "ISO 12156" {
        w1126 = "ISO 12156 TEST CONDITIONS" ("Standard 2")
        n916 = local write "Standard 2"(w1126) -> ()
        n917 = local write "Standard"(w1126) -> ()
      }
      frame "CEC F-096-A-06" {
        w1127 = "CEC F-096-A-06 TEST CONDITIONS" ("Standard 2")
        n918 = local write "Standard 2"(w1127) -> ()
        n919 = local write "Standard"(w1127) -> ()
      }
      frame "Custom" {
        w1128 = "CUSTOM TEST CONDITIONS" ("Standard 2")
        n920 = local write "Standard 2"(w1128) -> ()
        n921 = local write "Standard"(w1128) -> ()
      }
    }
    n922 = case shown="True" w891 {
      frame False {
        n923 = local write "Temperature On Command"(TRUE ("Temperature On Command")) -> ()
        n924 = case shown="True" "Temperature Off Command" {
          selector: "Temperature Off Command" -> [_ w1132]
          frame False {
          }
          frame True {
            n925 = Not(x=w1132) -> (.not. x?=w1131:bool)
            n926 = local read "EVENT LOG"() -> (w1135:string)
            n927 = local write "Temperature Off Command"(w1131) -> ()
            n928 = call "Event Log.vi"("Content"="Heater Off", "EVENT LOG"=w1135) -> ("EVENT LOG"=w1134:string)  [unwired: 8 in, 1 out]
            n929 = local write "EVENT LOG"(w1134) -> ()
          }
        }
      }
      frame True {
        n930 = local write "Temperature Off Command"(TRUE ("Temperature Off Command")) -> ()
        n931 = case shown="True" "Temperature On Command" {
          selector: "Temperature On Command" -> [_ w1139]
          frame False {
          }
          frame True {
            n932 = Not(x=w1139) -> (.not. x?=w1138:bool)
            n933 = local write "Temperature On Command"(w1138) -> ()
            n934 = disable-structure shown="Enabled" {
              disable-tunnel: "Heater On" -> [w1141 _]
              frame Enabled {
                n935 = local read "EVENT LOG"() -> (w1142:string)
                n936 = call "Event Log.vi"("Content"=w1141, "EVENT LOG"=w1142) -> ("EVENT LOG"=w1143:string)  [unwired: 8 in, 1 out]
                n937 = local write "EVENT LOG"(w1143) -> ()
              }
              frame Disabled {
              }
            }
          }
        }
      }
    }
    n938 = local read "Main Tab"() -> (w882:T2)
    n939 = case shown="\"About\"" w882 {
      frame "HOME", Default {
        w928 = T15."Enabled" ("Disabled")
        n940 = local read "Service Password enable"() -> (w927:bool)
        n941 = property on="Imaging" class="Bool (strict)"("DisabledEnum"=w928) -> ()  [unwired: 2 in, 2 out]
        n942 = property on="Dashboard" class="Bool (strict)"("DisabledEnum"=w928) -> ()  [unwired: 2 in, 2 out]
        n943 = property on="Test Setup" class="Bool (strict)"("DisabledEnum"=w928) -> ()  [unwired: 2 in, 2 out]
        n944 = property on="Analysis" class="Bool (strict)"("DisabledEnum"=w928) -> ()  [unwired: 2 in, 2 out]
        n945 = property on="Home" class="Bool (strict)"("DisabledEnum"=w928) -> ()  [unwired: 2 in, 2 out]
        n946 = property on="Report" class="Bool (strict)"("DisabledEnum"=w928) -> ()  [unwired: 2 in, 2 out]
        n947 = property on="Main Dashboard Buttons" class="RadioBtnsControl (strict)"("DisabledEnum"=w928) -> ()  [unwired: 2 in, 2 out]
        n948 = case shown="True" w927 {
          tunnel: [T15."Disabled" ("Disabled") T15."Enabled" ("Disabled")] -> w926
          frame False {
          }
          frame True {
          }
        }
        n949 = property on="About" class="Bool (strict)"("DisabledEnum"=w926) -> ()  [unwired: 2 in, 2 out]
      }
      frame "Test Setup" {
        w933 = T15."Enabled" ("Disabled")
        n950 = local read "Service Password enable"() -> (w932:bool)
        n951 = property on="Dashboard" class="Bool (strict)"("DisabledEnum"=T15."Disabled" ("Disabled")) -> ()  [unwired: 2 in, 2 out]
        n952 = property on="Imaging" class="Bool (strict)"("DisabledEnum"=w933) -> ()  [unwired: 2 in, 2 out]
        n953 = property on="Analysis" class="Bool (strict)"("DisabledEnum"=w933) -> ()  [unwired: 2 in, 2 out]
        n954 = property on="Home" class="Bool (strict)"("DisabledEnum"=w933) -> ()  [unwired: 2 in, 2 out]
        n955 = property on="Report" class="Bool (strict)"("DisabledEnum"=w933) -> ()  [unwired: 2 in, 2 out]
        n956 = property on="Test Setup" class="Bool (strict)"("DisabledEnum"=w933) -> ()  [unwired: 2 in, 2 out]
        n957 = case shown="True" w932 {
          tunnel: [T15."Disabled" ("Disabled") T15."Enabled" ("Disabled")] -> w931
          frame False {
          }
          frame True {
          }
        }
        n958 = property on="About" class="Bool (strict)"("DisabledEnum"=w931) -> ()  [unwired: 2 in, 2 out]
      }
      frame "Adv Scar" {
        w940 = T15."Enabled" ("Disabled")
        n959 = property on="Dashboard" class="Bool (strict)"("DisabledEnum"=T15."Disabled" ("Disabled")) -> ()  [unwired: 2 in, 2 out]
        n960 = property on="Imaging" class="Bool (strict)"("DisabledEnum"=w940) -> ()  [unwired: 2 in, 2 out]
        n961 = property on="Analysis" class="Bool (strict)"("DisabledEnum"=w940) -> ()  [unwired: 2 in, 2 out]
        n962 = property on="Home" class="Bool (strict)"("DisabledEnum"=w940) -> ()  [unwired: 2 in, 2 out]
        n963 = property on="Report" class="Bool (strict)"("DisabledEnum"=w940) -> ()  [unwired: 2 in, 2 out]
        n964 = property on="Test Setup" class="Bool (strict)"("DisabledEnum"=w940) -> ()  [unwired: 2 in, 2 out]
        n965 = local read "Service Password enable"() -> (w938:bool)
        n966 = case shown="True" w938 {
          tunnel: [T15."Disabled" ("Disabled") T15."Enabled" ("Disabled")] -> w937
          frame False {
          }
          frame True {
          }
        }
        n967 = property on="About" class="Bool (strict)"("DisabledEnum"=w937) -> ()  [unwired: 2 in, 2 out]
      }
      frame "Adv Scar Report" {
        w945 = T15."Enabled" ("Disabled")
        n968 = property on="Dashboard" class="Bool (strict)"("DisabledEnum"=T15."Disabled" ("Disabled")) -> ()  [unwired: 2 in, 2 out]
        n969 = property on="Imaging" class="Bool (strict)"("DisabledEnum"=w945) -> ()  [unwired: 2 in, 2 out]
        n970 = property on="Analysis" class="Bool (strict)"("DisabledEnum"=w945) -> ()  [unwired: 2 in, 2 out]
        n971 = property on="Home" class="Bool (strict)"("DisabledEnum"=w945) -> ()  [unwired: 2 in, 2 out]
        n972 = property on="Report" class="Bool (strict)"("DisabledEnum"=w945) -> ()  [unwired: 2 in, 2 out]
        n973 = property on="Test Setup" class="Bool (strict)"("DisabledEnum"=w945) -> ()  [unwired: 2 in, 2 out]
        n974 = local read "Service Password enable"() -> (w944:bool)
        n975 = case shown="True" w944 {
          tunnel: [T15."Disabled" ("Disabled") T15."Enabled" ("Disabled")] -> w943
          frame False {
          }
          frame True {
          }
        }
        n976 = property on="About" class="Bool (strict)"("DisabledEnum"=w943) -> ()  [unwired: 2 in, 2 out]
      }
      frame "Compare Files" {
        w951 = T15."Enabled" ("Disabled")
        n977 = local read "Service Password enable"() -> (w950:bool)
        n978 = property on="Dashboard" class="Bool (strict)"("DisabledEnum"=T15."Disabled" ("Disabled")) -> ()  [unwired: 2 in, 2 out]
        n979 = property on="Imaging" class="Bool (strict)"("DisabledEnum"=w951) -> ()  [unwired: 2 in, 2 out]
        n980 = property on="Analysis" class="Bool (strict)"("DisabledEnum"=w951) -> ()  [unwired: 2 in, 2 out]
        n981 = property on="Home" class="Bool (strict)"("DisabledEnum"=w951) -> ()  [unwired: 2 in, 2 out]
        n982 = property on="Report" class="Bool (strict)"("DisabledEnum"=w951) -> ()  [unwired: 2 in, 2 out]
        n983 = property on="Test Setup" class="Bool (strict)"("DisabledEnum"=w951) -> ()  [unwired: 2 in, 2 out]
        n984 = case shown="True" w950 {
          tunnel: [T15."Disabled" ("Disabled") T15."Enabled" ("Disabled")] -> w949
          frame False {
          }
          frame True {
          }
        }
        n985 = property on="About" class="Bool (strict)"("DisabledEnum"=w949) -> ()  [unwired: 2 in, 2 out]
      }
      frame "Acquire" {
        n986 = local read "Service Password enable"() -> (w955:bool)
        n987 = property on="Test Setup" class="Bool (strict)"("DisabledEnum"=T15."Disabled" ("Disabled")) -> ()  [unwired: 2 in, 2 out]
        n988 = local read "Auto Start Test"() -> (w957:bool)
        n989 = local read "RUN"() -> (w959:bool)
        n990 = case shown="True" w955 {
          tunnel: [T15."Disabled" ("Disabled") T15."Enabled" ("Disabled")] -> w956
          frame False {
          }
          frame True {
          }
        }
        n991 = Or(x=w959, y=w957) -> (x .or. y?=w958:bool)
        n992 = case shown="True" w958 {
          tunnel: [T15."Enabled" ("Disabled") T15."Disabled" ("Disabled")] -> w961
          frame False {
          }
          frame True {
          }
        }
        n993 = property on="About" class="Bool (strict)"("DisabledEnum"=w956) -> ()  [unwired: 2 in, 2 out]
        n994 = property on="Imaging" class="Bool (strict)"("DisabledEnum"=w961) -> ()  [unwired: 2 in, 2 out]
        n995 = property on="Dashboard" class="Bool (strict)"("DisabledEnum"=w961) -> ()  [unwired: 2 in, 2 out]
        n996 = property on="Analysis" class="Bool (strict)"("DisabledEnum"=w961) -> ()  [unwired: 2 in, 2 out]
        n997 = property on="Home" class="Bool (strict)"("DisabledEnum"=w961) -> ()  [unwired: 2 in, 2 out]
        n998 = property on="Report" class="Bool (strict)"("DisabledEnum"=w961) -> ()  [unwired: 2 in, 2 out]
      }
      frame "About" {
        n999 = local read "FILE"() -> (w973:string)
        n1000 = local read "TEST FILE NAM,E SAVED"() -> (w966:bool)
        n1001 = call <vilib>:"Trim Whitespace.vi"("string"=w973) -> ("trimmed string"=w972:string)  [unwired: 1 in]
        n1002 = local read "Auto Start Test"() -> (w976:bool)
        n1003 = String Length(string=w972) -> (length=w971:i32)
        n1004 = Greater?(x=w971, y=1) -> (0:w968:bool)
        n1005 = And(x=w968, y=w966) -> (x .and. y?=w967:bool)
        n1006 = local read "RUN"() -> (w978:bool)
        n1007 = case shown="True" w967 {
          tunnel: [T15."Disabled" ("Disabled") T15."Enabled" ("Disabled")] -> w969
          frame False {
          }
          frame True {
          }
        }
        n1008 = Or(x=w978, y=w976) -> (x .or. y?=w977:bool)
        n1009 = property on="About" class="Bool (strict)"("DisabledEnum"=T15."Enabled" ("Disabled")) -> ()  [unwired: 2 in, 2 out]
        n1010 = case shown="True" w977 {
          tunnel: [T15."Enabled" ("Disabled") T15."Disabled" ("Disabled")] -> w975
          frame False {
          }
          frame True {
          }
        }
        n1011 = property on="Dashboard" class="Bool (strict)"("DisabledEnum"=w969) -> ()  [unwired: 2 in, 2 out]
        n1012 = property on="Test Setup" class="Bool (strict)"("DisabledEnum"=w975) -> ()  [unwired: 2 in, 2 out]
        n1013 = property on="Imaging" class="Bool (strict)"("DisabledEnum"=w975) -> ()  [unwired: 2 in, 2 out]
        n1014 = property on="Analysis" class="Bool (strict)"("DisabledEnum"=w975) -> ()  [unwired: 2 in, 2 out]
        n1015 = property on="Home" class="Bool (strict)"("DisabledEnum"=w975) -> ()  [unwired: 2 in, 2 out]
        n1016 = property on="Report" class="Bool (strict)"("DisabledEnum"=w975) -> ()  [unwired: 2 in, 2 out]
      }
    }
    n1017 = local read "Quit"() -> (w910:bool)
    "Single" <- "Single - Graph"
  }
  n1018 = disable-structure shown="Disabled" {
    disable-tunnel: [w1218 _] -> w31
    disable-tunnel: _ -> [w1217 _]
    frame Disabled {
      n1019 = while {
        tunnel: w1217 -> [_]
        tunnel: [w1219] -> w1218
        tunnel: [w1220] -> _
        i -> [w1220]
        stop <- w1219 stop-if-true
        w1236 = u16 10 items=["1.0"=10, "1.5"=15, "2.0"=20] ("stop bits (10: 1 bit)")
        n1020 = Wait (ms)(milliseconds to wait=u32 10) -> ()  [unwired: 1 out]
